vi "Encoder Angles.vi"(8 "calibration angle":dbl, 9 "low voltage":dbl, 10 "top voltage":dbl, 11 "AIDeviceRef Encoder":T1={"DevStatus"={"status"=FALSE, "code"=0, "source"=""}, "Controller"=enum."Controller 1", "Analog Channel"=enum."AI 1"}) -> (3 "encoder angle":dbl)   [LabVIEW 2014]
uses:
  <vilib>/Rock Robotics/WPI/AnalogChannel/WPI_AnalogChannelDevRef.ctl
  <vilib>/Rock Robotics/SystemInterfaces/Typedef/FPGA_TypedefAnalogModule.ctl
  <vilib>/Rock Robotics/SystemInterfaces/AI/FPGA_AIChannel.ctl
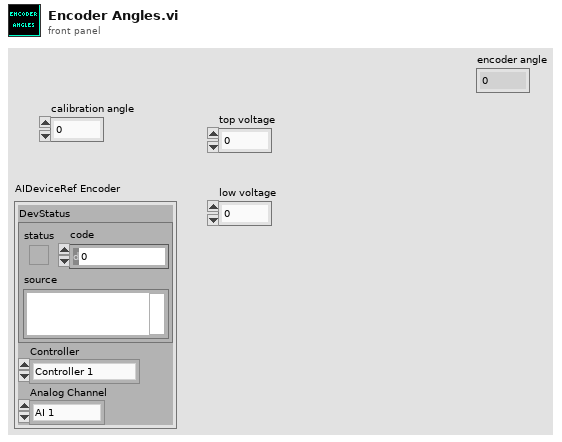
[diagram p1: front panel]
types:
  T1 = typedef "WPI_AnalogChannelDevRef.ctl" = cluster{"DevStatus":errorcluster, "Controller":T2, "Analog Channel":T3}
  T2 = typedef "FPGA_TypedefAnalogModule.ctl" = enum16{"Controller 1"}
  T3 = typedef "FPGA_AIChannel.ctl" = enum8{"AI 0", "AI 1", "AI 2", "AI 3", "AI MXP 0", "AI MXP 1", "AI MXP 2", "AI MXP 3", "Invalid"}
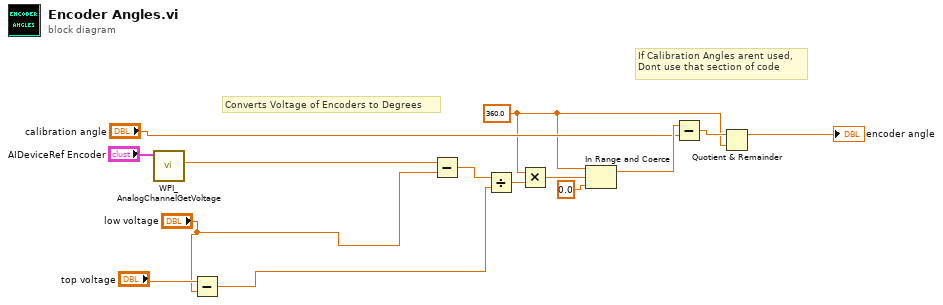
[diagram p0: block diagram]
diagram:
  w3 = 360.0 ("y")
  # "Converts Voltage of Encoders to Degrees"
  # "If Calibration Angles arent used,\nDont use that section of code"
  n1 = call <vilib>:"WPI_AnalogChannelGetVoltage.vi"("AIDeviceRef"="AIDeviceRef Encoder") -> ("Voltage"=w1:dbl)  [unwired: 8 in, 2 out]
  n2 = Subtract(x="top voltage", y="low voltage") -> (x-y=w8:dbl)
  n3 = Subtract(x=w1, y="low voltage") -> (x-y=w14:dbl)
  n4 = Divide(x=w14, y=w8) -> (x/y=w13:dbl)
  n5 = Multiply(x=w3, y=w13) -> (x*y=w12:dbl)
  n6 = In Range and Coerce(upper limit=w3, x=w12, lower limit=0.0) -> (coerced(x)=w6:dbl)  [unwired: 1 out]
  n7 = Subtract(x=w6, y="calibration angle") -> (x-y=w4:dbl)
  n8 = Quotient & Remainder(x=w4, y=w3) -> (x-y*floor(x/y)=→"encoder angle":dbl)  [unwired: 1 out]
